vi "Select pin on PCB.vi"(0 "Pin":dbl, 3 "error in":errorcluster) -> (10 "error out":errorcluster)   [LabVIEW 2011]
uses:
  <vilib>/ULx/Create Channel.llb/ULx Create Channel (DO-Digital Output).vi
  <vilib>/ULx/Write.llb/ULx Write (Digital U32 1Chan 1Samp).vi
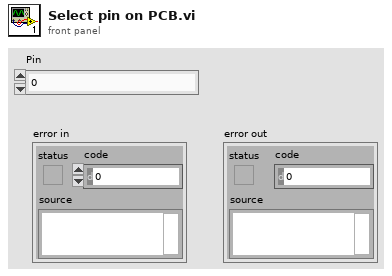
[diagram p1: front panel]
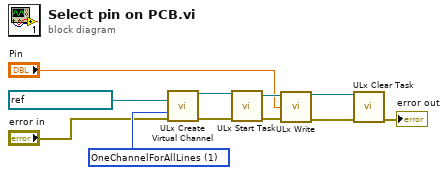
[diagram p0: block diagram]
diagram:
  w11 = 1 items=["OneChannelForEachLine", "OneChannelForAllLines"] ("line grouping")
  n1 = call-poly <vilib>:"ULx Create Virtual Channel.vi"("lines"=refnum<k21> "Dev0/1stPortA" ("Port 2"), "line grouping"=w11, "error in"="error in") -> ("task out"=w9:refnum<k24>, "error out"=w10:errorcluster)  [unwired: 11 in]
  n2 = call <vilib>:"ULx Start Task.vi"("task in"=w9, "error in"=w10) -> ("task out"=w6:refnum<k24>, "error out"=w5:errorcluster)  [unwired: 12 in]
  n3 = call-poly <vilib>:"ULx Write.vi"("task in"=w6, "data"="Pin", "error in"=w5) -> ("task out"=w8:refnum<k24>, "error out"=w7:errorcluster)  [unwired: 10 in, 1 out]
  n4 = call <vilib>:"ULx Clear Task.vi"("task in"=w8, "error in"=w7) -> ("error out"=→"error out":errorcluster)  [unwired: 13 in]
